vi "Set View by Tab Index.vi"(8 "error in (no error)":errorcluster, 10 "Index":i32, 11 "TabbedViewManager In":refnum<class "TabbedViewManager.lvclass">) -> (0 "error out":errorcluster, 3 "TabbedViewManager Out":refnum<class "TabbedViewManager.lvclass">)   [LabVIEW 2015, in "TabbedViewManager.lvlib" / "TabbedViewManager.lvclass"]
uses:
  TabbedViewManager.lvclass
  Framework/IViewManager/IViewManager/IViewManager.lvclass/IViewManager.ctl
  TabbedViewManager.lvclass/TabbedViewManager.ctl
  Framework/IViewable/IViewable Messages/Insert View Msg/Insert View Msg.lvclass/Insert View Msg.ctl
  <vilib>/ActorFramework/Message Enqueuer/Message Enqueuer.lvclass/Message Enqueuer.ctl
  <vilib>/ActorFramework/Message Enqueuer/Enqueue.vi
  <vilib>/ActorFramework/Message Priority Queue/Priority Enqueue.vi
  Framework/IViewable/IViewable Messages/Insert View Msg/Insert View Msg.lvclass
  Framework/IViewManager/IViewManager/IViewManager.lvclass
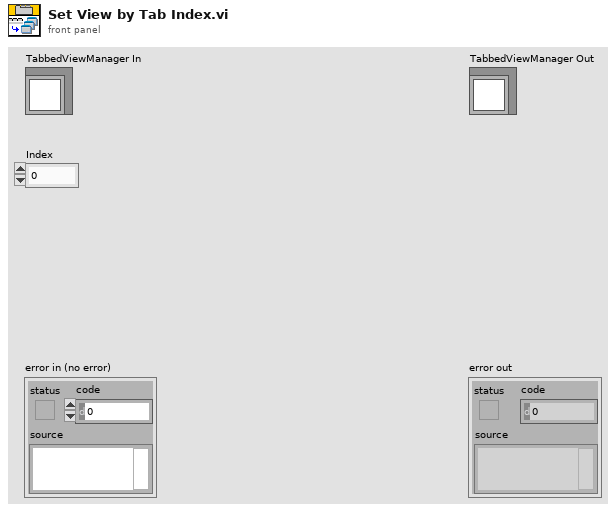
[diagram p1: front panel]
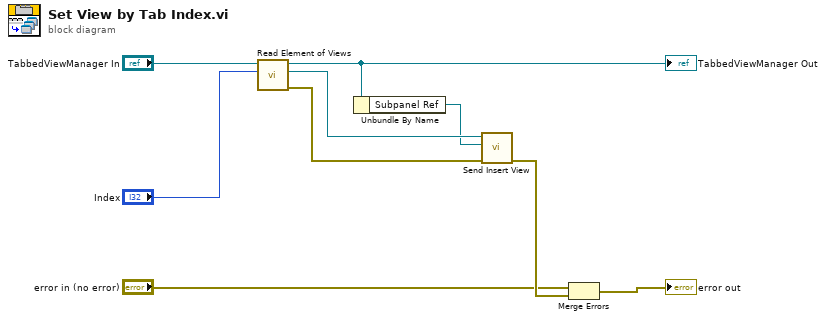
[diagram p0: block diagram]
diagram:
  n1 = call "Read Element of Views.vi"("Index"="Index", "IViewManager In"="TabbedViewManager In") -> ("error out"=w4:errorcluster, "View Ref"=w5:refnum<class "Message Enqueuer.lvclass">, "IViewManager Out"=w7:refnum<class "TabbedViewManager.lvclass">)  [unwired: 7 in]
  "TabbedViewManager Out" <- w7
  n2 = Unbundle By Name(w7) -> ("Subpanel Ref"=w3:refnum<vi>)
  n3 = call "Send Insert View.vi"("error in (no error)"=w4, "SubPnl Refnum"=w3, "Message Enqueuer"=w5) -> ("error out"=w9:errorcluster)  [unwired: 7 in, 1 out]
  n4 = Merge Errors("error in (no error)", w9) -> (→"error out":errorcluster)
